vi "PRO_Check Resistor.vi"(8 "Results In in":T2 {"Resistor" format="%.1f"; "Drain" format="%.3f"; "Fill" format="%.3f"}, 9 "Full Cfg":T3, 10 "Measurement":T1, 11 "ChA/!ChB":bool) -> (0 "Results In out":T2 {"Resistor" format="%.1f"; "Drain" format="%.3f"; "Fill" format="%.3f"})   [LabVIEW 2024]
uses:
  Control Definitions/Def FullCfg.ctl
  Control Definitions/Def BenchCfg.ctl
  Control Definitions/Def PumpCtlRefs.ctl
  Control Definitions/Def Bench Status.ctl
  Control Definitions/Def Results2.ctl
  Control Definitions/Def Xresult.ctl
panel:
  out "error in (no error)":errorcluster
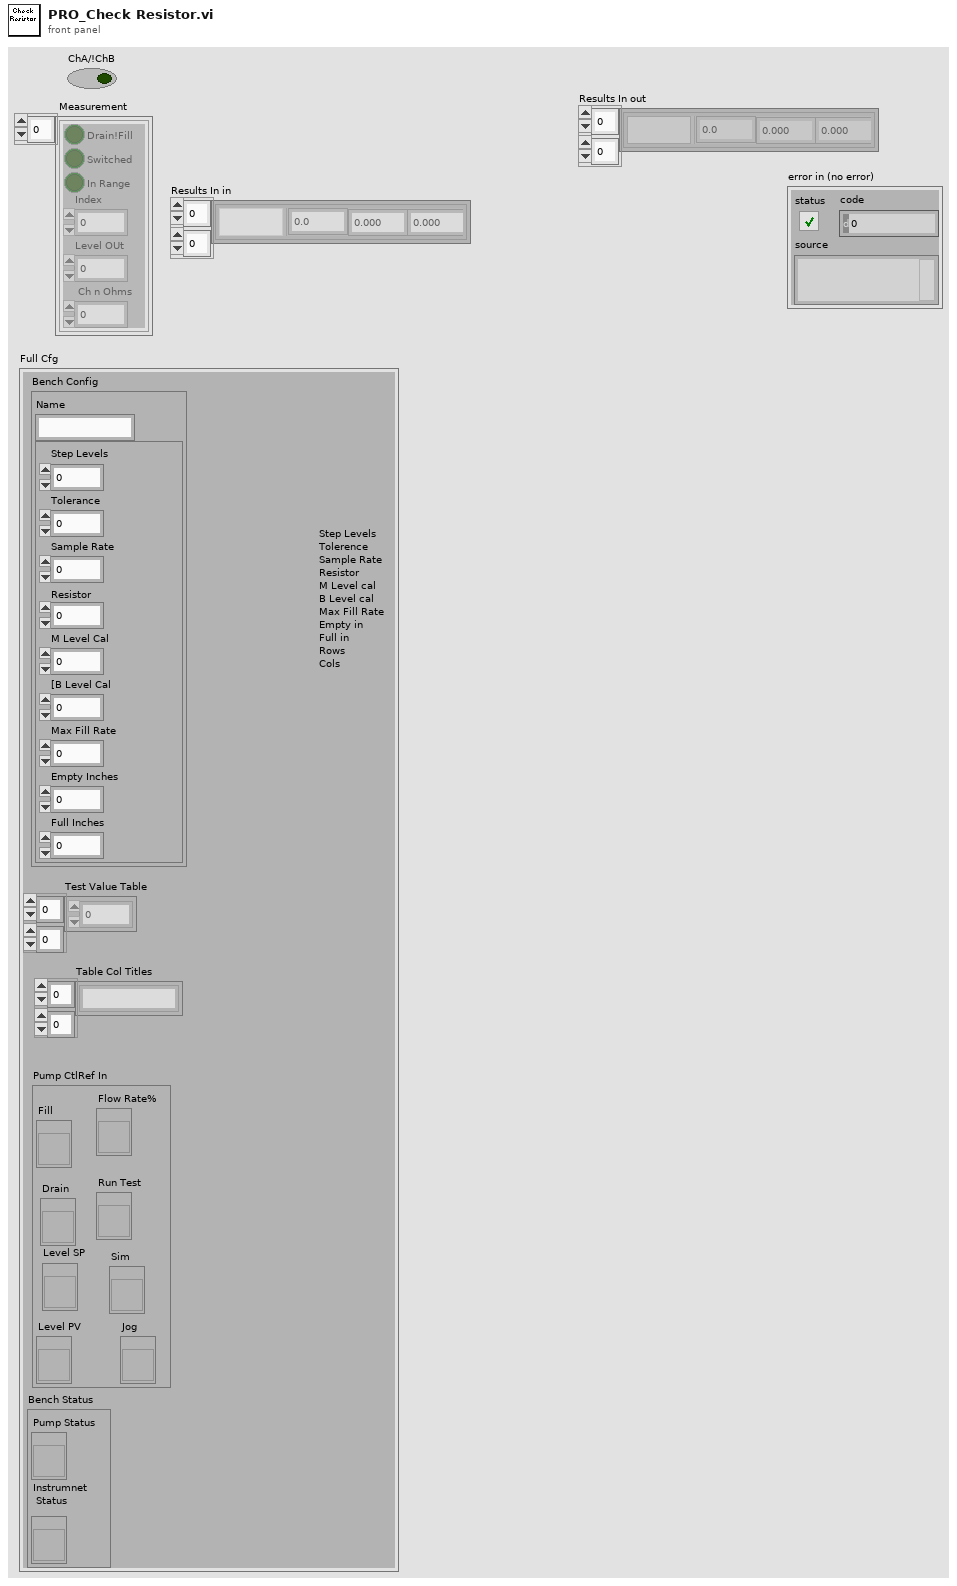
[diagram p1: front panel]
types:
  T1 = typedef "Def Xresult.ctl" = cluster{"Switched":bool, "In Range":bool, "Index":i16, "Level OUt":dbl, " Ch n Ohms":dbl, "Drain!Fill":bool}[]
  T2 = typedef "Def Results2.ctl" = cluster{"Fill":dbl, "Drain":dbl, "Status":i16, "Resistor":dbl}[][]
  T3 = typedef "Def FullCfg.ctl" = cluster{"Bench Config":T4, "Test Value Table ":dbl[][], "Table Col Titles":string[][], "Pump CtlRef In":T5, "Bench Status":T6}
  T4 = typedef "Def BenchCfg.ctl" = cluster{"Name":string, cluster{"Step Levels":dbl, "Tolerance":dbl, "Sample Rate":dbl, "Resistor":dbl, "M Level Cal":dbl, "[B Level Cal":dbl, "Max Fill Rate":dbl, "Empty Inches":dbl, "Full Inches":dbl}}
  T5 = typedef "Def PumpCtlRefs.ctl" = cluster{"Fill ":refnum<vi>, "Drain":refnum<vi>, "Level PV":refnum<vi>, "Flow Rate%":refnum<vi>, "Run Test":refnum<vi>, "Sim":refnum<vi>, "Jog":refnum<vi>, "Level SP":refnum<vi>}
  T6 = typedef "Def Bench Status.ctl" = cluster{"Pump Status":refnum<vi>, "Instrumnet\n Status":refnum<vi>}
  T7 = cluster{"Switched":bool, "In Range":bool, "Index":i16, "Level OUt":dbl, " Ch n Ohms":dbl, "Drain!Fill":bool}
  T8 = typedef "Ded Spec RNG.ctl" = cluster{"Status":cluster{"ChA/!ChB":bool, "Drain/!Fill":bool, "In Range?":bool, "Switch Range?":bool, "Measure R?":bool}, "Specs":dbl[], "Indes":i32}
  T9 = cluster{"Fill":dbl, "Drain":dbl, "Status":i16, "Resistor":dbl}
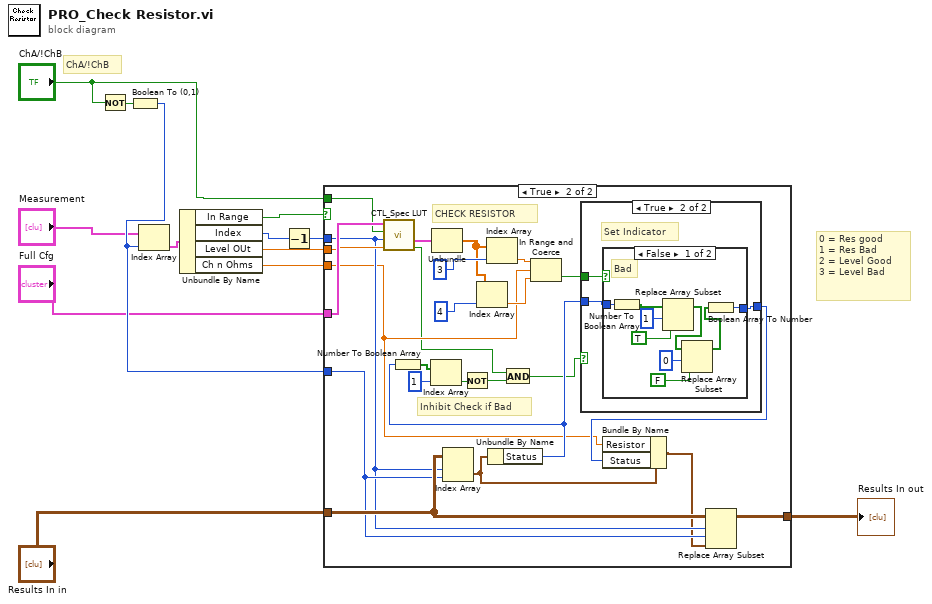
[diagram p0: block diagram]
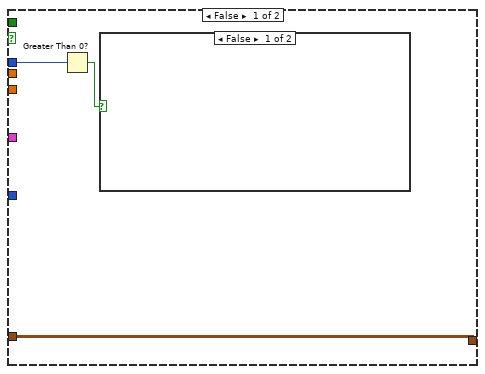
[diagram p2: hidden frame]
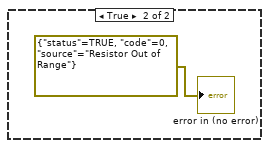
[diagram p3: hidden frame]
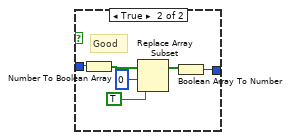
[diagram p5: hidden frame]
diagram:
  # "0 = Res good\n1 = Res Bad\n2 = Level Good\n3 = Level Bad"
  # "ChA/!ChB"
  n1 = Not(x="ChA/!ChB") -> (.not. x?=w12:bool)
  n2 = Boolean To (0,1)(Boolean=w12) -> (0, 1=w13:i16)
  n3 = Index Array(array="Measurement", index=w13) -> (element=w3:T7)
  n4 = Unbundle By Name(w3) -> ("In Range"=w7:bool, "Index"=w10:i16, "Level OUt"=w5:dbl, "Ch n Ohms"=w6:dbl)
  n5 = Decrement(x=w10) -> (x-1=w9:i16)
  n6 = case shown="True" w7 {
    tunnel: "Full Cfg" -> [_ w39]
    tunnel: [w16 w42] -> w1
    tunnel: "Results In in" -> [w16 w41]
    tunnel: w5 -> [_ w32]
    tunnel: w6 -> [_ w21]
    tunnel: w13 -> [_ w40]
    tunnel: w9 -> [w15 w31]
    tunnel: "ChA/!ChB" -> [_ w38]
    frame False {
      n7 = Greater Than 0?(x=w15) -> (x > 0?=w14:bool)
      n8 = case shown="False" w14 {
        frame False {
        }
        frame True {
          "error in (no error)" <- errorcluster {"status"=TRUE, "code"=0, "source"="Resistor Out of Range"} ("error in (no error)")
        }
      }
    }
    frame True {
      # "CHECK RESISTOR"
      # "Inhibit Check if Bad"
      n9 = call "CTL_Spec LUT.vi"("Level IN inches"=w32, "Index"=w31, "ChA/!ChB"=w38, "Full Cfg"=w39) -> ("Res In Range?"=w20:bool, "Spec RNG"=w37:T8)  [unwired: 4 in, 2 out]
      n10 = Unbundle(w37) -> ("Specs"=w18:dbl[])  [unwired: 2 out]
      n11 = Index Array(array=w41, index (row)=w31, index (col)=w40) -> (element=w30:T9)
      n12 = Index Array(array=w18, index=4) -> (element=w33:dbl)
      n13 = Index Array(array=w18, index=3) -> (element=w34:dbl)
      n14 = Unbundle By Name(w30) -> ("Status"=w26:i16)
      n15 = Number To Boolean Array(number=w26) -> (Boolean array=w25:bool[])
      n16 = Index Array(array=w25, index=1) -> (element=w23:bool)
      n17 = Not(x=w23) -> (.not. x?=w22:bool)
      n18 = And(x=w20, y=w22) -> (x .and. y?=w19:bool)
      n19 = In Range and Coerce(upper limit=w34, x=w21, lower limit=w33) -> (In Range?=w27:bool)  [unwired: 1 out]
      n20 = case shown="True" w19 {
        tunnel: w26 -> [w43 w46]
        tunnel: [w43 w45] -> w28
        tunnel: w27 -> [_ w44]
        frame False {
          # "Out of Range \nDon't Change"
        }
        frame True {
          # "Set Indicator"
          n21 = case shown="False" w44 {
            tunnel: w46 -> [w53 w61]
            tunnel: [w51 w58] -> w45
            frame False {
              # "Bad"
              n22 = Number To Boolean Array(number=w53) -> (Boolean array=w52:bool[])
              n23 = Replace Array Subset(array=w52, new element=TRUE ("new element/subarray"), index=1) -> (w48:bool[])
              n24 = Replace Array Subset(array=w48, new element=FALSE ("new element/subarray"), index=0) -> (w47:bool[])
              n25 = Boolean Array To Number(Boolean array=w47) -> (number=w51:u32)
            }
            frame True {
              # "Good"
              n26 = Number To Boolean Array(number=w61) -> (Boolean array=w60:bool[])
              n27 = Replace Array Subset(array=w60, new element=TRUE ("new element/subarray"), index=0) -> (w59:bool[])
              n28 = Boolean Array To Number(Boolean array=w59) -> (number=w58:u32)
            }
          }
        }
      }
      n29 = Bundle By Name(cluster=w30, "Resistor"=w21, "Status"=w28) -> (w29:T9)
      n30 = Replace Array Subset(array=w41, new element=w29, index (row)=w31, index (col)=w40) -> (w42:T2)
    }
  }
  "Results In out" <- w1
